vi "CSM - Refesh More Template Palette.vi"   [LabVIEW 2014]
uses:
  <vilib>/Palette API/Palette Menu/Public Type Define/Palette type.ctl
  <vilib>/Palette API/Palette Menu/Public Type Define/Item.ctl
  <vilib>/Palette API/Palette Menu/Palette Menu.lvlib
types:
  T1 = typedef "Palette Menu.lvlib/Palette type.ctl" = i32
  T2 = typedef "Palette Menu.lvlib/Palette Data.ctl" = cluster{"display name":string, "view format":T3, "palette width":i16, "items":T4, "256 color icon":picture, "B&W color icon":picture, "help information":T6, "palette description":string, "synchronize information":T7}
  T3 = typedef "Palette Menu.lvlib/View Format.ctl" = u16
  T4 = typedef "Palette Menu.lvlib/Items.ctl" = T5[]
  T5 = typedef "Palette Menu.lvlib/Item.ctl" = cluster{"item path":path, "library path (.lvlib)":path, "use default lvlib palette":bool, "short name":string, "place VI contents":bool, "hide synchronized item":bool, "reserve spot for synch item":bool, "configure when placing VI contents":bool}
  T6 = typedef "Palette Menu.lvlib/Help Info.ctl" = cluster{"help tag":string, "help file path ":path}
  T7 = typedef "Palette Menu.lvlib/Synchronize Info.ctl" = cluster{"synchronize with directory":bool, "synchronize directory path":path}
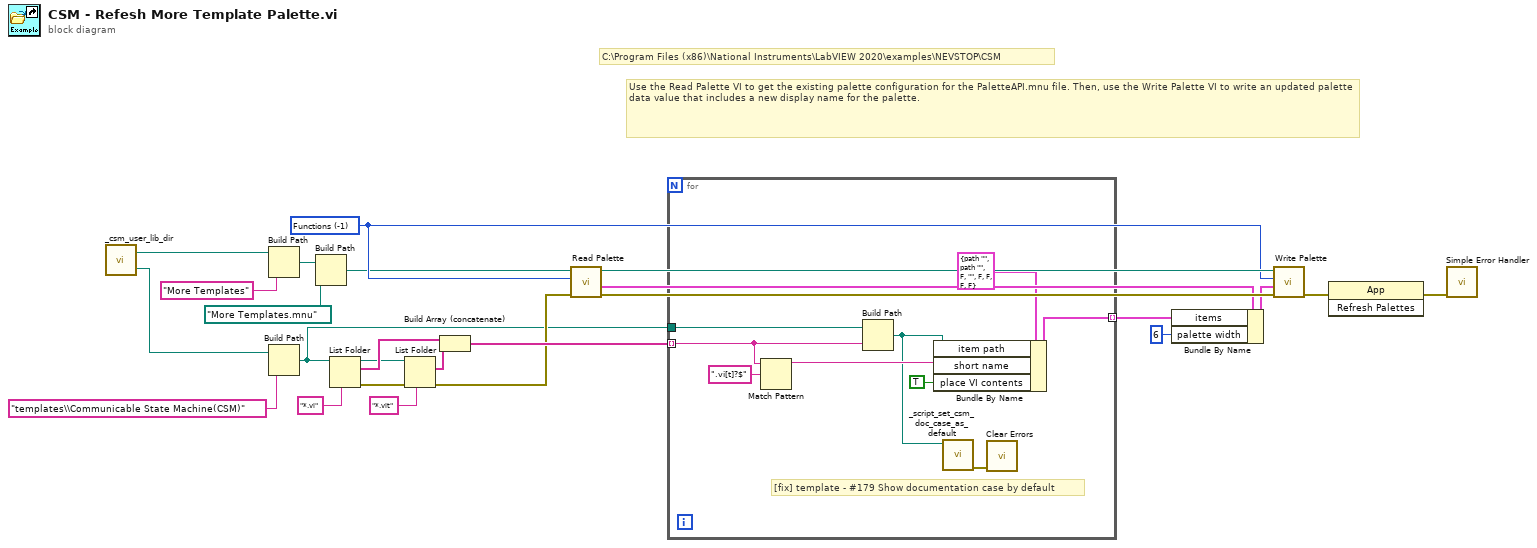
[diagram p0: block diagram]
diagram:
  w23 = T1 -1 items=["Functions"=-1, "Controls"=-2] ("palette type")
  # "Use the Read Palette VI to get the existing palette configuration for the PaletteAPI.mnu file. Then, use the Write Palette VI to write an updated palette data value that includes a new display name for the palette."
  # "C:\\Program Files (x86)\\National Instruments\\LabVIEW 2020\\examples\\NEVSTOP\\CSM"
  n1 = call "_csm_user_lib_dir.vi"() -> ("<LabVIEW>"=w2:path, "csm_user.lib_dir"=w13:path)  [unwired: 2 in]
  n2 = Build Path(base path=w13, name or relative path="More Templates") -> (appended path=w15:path)
  n3 = Build Path(base path=w2, name or relative path="templates\\Communicable State Machine(CSM)") -> (appended path=w4:path)
  n4 = Build Path(base path=w15, name or relative path=path "More Templates.mnu") -> (appended path=w22:path)
  n5 = List Folder(path=w4, pattern="*.vi") -> (path out=w3:path, filenames=w9:string[], error out=w10:errorcluster)  [unwired: 2 in, 1 out]
  n6 = List Folder(path=w3, pattern="*.vit", error in=w10) -> (filenames=w8:string[], error out=w5:errorcluster)  [unwired: 1 in, 2 out]
  n7 = Build Array (concatenate)(w9, w8) -> (w6:string[])
  n8 = call <vilib>:"Read Palette.vi"("error in (no error)"=w5, "palette type"=w23, "palette path"=w22) -> ("error out"=w25:errorcluster, "palette data"=w20:T2, "duplicate palette path"=w24:path)  [unwired: 1 in, 5 out]
  n9 = for {
    tunnel: [w34] -> w7 mode=indexing
    tunnel: w6 -> [w30] mode=indexing
    tunnel: w4 -> [w31]
    # "[fix] template - #179 Show documentation case by default"
    n10 = Match Pattern(string=w30, regular expression=".vi[t]?$") -> (before substring=w28:string)  [unwired: 1 in, 3 out]
    n11 = Build Path(base path=w31, name or relative path=w30) -> (appended path=w26:path)
    n12 = Bundle By Name(cluster=T5 {"item path"=path "", "library path (.lvlib)"=path "", "use default lvlib palette"=FALSE, "short name"="", "place VI contents"=FALSE, "hide synchronized item"=FALSE, "reserve spot for synch item"=FALSE, "configure when placing VI contents"=FALSE} ("Items"), "item path"=w26, "short name"=w28, "place VI contents"=TRUE) -> (w34:T5)
    n13 = call "_script_set_csm_doc_case_as_default.vi"("vi path"=w26) -> ("error out"=w27:errorcluster)  [unwired: 10 in]
    n14 = call <vilib>:"Clear Errors.vi"("error in (no error)"=w27) -> ()  [unwired: 6 in, 1 out]
  }
  n15 = Bundle By Name(cluster=w20, "items"=w7, "palette width"=i16 6) -> (w19:T2)
  n16 = call <vilib>:"Write Palette.vi"("error in (no error)"=w25, "palette data"=w19, "palette type"=w23, "palette path"=w24) -> ("error out"=w17:errorcluster)  [unwired: 1 in, 6 out]
  n17 = invoke class="App" method="Refresh Palettes"(error in=w17) -> (error out=w18:errorcluster)  [unwired: 2 in, 2 out]
  n18 = call <vilib>:"Simple Error Handler.vi"("error in (no error)"=w18) -> ()  [unwired: 1 in, 8 out]
